vi "JSON to Cluster.vi"(5 "JSON":string, 6 "JSONtext LVClass Serializer in":refnum<class "JSONtext LVClass Serializer.lvclass">, 7 "Item Offset":i32, 8 "error in (no error)":errorcluster, 9 "Element Info":T3(array[cluster]), 10 "Elements":variant[](array[variant]), 11 "ELement Names (as JSON)":string[](array[string])) -> (0 "error out":errorcluster, 3 "Cluster of Variants":variant)   [LabVIEW 2024, in "JSONtext.lvlib"]
uses:
  JSONtext.lvlib
  JSONtext LVClass Serializer.lvclass
  Data Type.ctl
  Tag Type.ctl
  Advance past whitespace.vi
  Commas Needed.vi
  Advance past whitespace and comma.vi
  Advance past next JSON Value (inlined COPY).vi
  Advance past Item Name.vi
  Advance past Line Ending.vi
  Advance past String.vi
  Advance past Number.vi
  Error Cluster From Error Code.vi
  Advance past Array.vi
  Advance past Object.vi
  Parsing Error.vi
  JDP Utility.lvlib
  NI_Data Type.lvlib
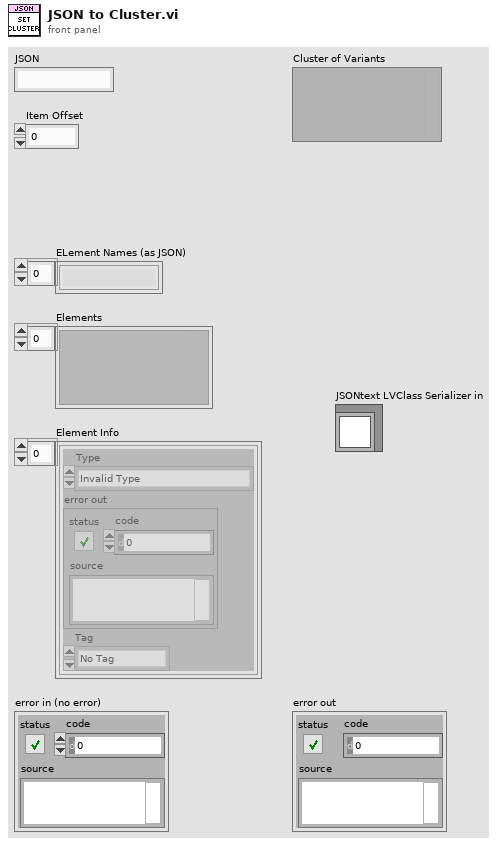
[diagram p1: front panel]
types:
  T1 = typedef "NI_Data Type.lvlib/Data Type.ctl" = enum8{"Invalid Type", "Void", "I8", "I16", "I32", "I64", "U8", "U16", "U32", "U64", "Single Float", "Double Float", "Extended Float", "Single Complex", "Double Complex", "Extended Complex", "Enum U8", "Enum U16", "Enum U32", "Enum U64", "Single Float With Unit", "Double Float With Unit", "Extended Float With Unit", "Single Complex with Unit", "Double Complex with Unit", "Extended Complex with Unit", "Boolean", "String", "Path", "Picture", "Tag", "Array", "Cluster", "Variant", "LV Variant", "Waveform", "Timestamp", "Digital Waveform", "Digital Data", "ExpressData", "Refnum", "External Data", "VI", "Poly VI", "LabVIEW Class Instance", "Fixed Point", "Set Collection", "Map Collection"}
  T2 = typedef "JSONtext.lvlib/Tag Type.ctl" = enum16{"No Tag", "<JSON>", "<JOBJ>", "<UTF8>"}
  T3 = cluster{"Type":T1, "error out":errorcluster, "Tag":T2}[]
  T4 = typedef "JSONtext.lvlib/JSON Value Type.ctl" = enum16{"Not a JSON Value", "JSON Object", "JSON Array", "String", "Number", "true", "false", "null"}
  T5 = typedef "JSONtext.lvlib/Found Items.ctl" = cluster{"Item offset":i32, "Offset past Item":i32, "Name offset":i32, "Offset past Name":i32, "Found":bool, "Item Type":T6, "Item Index":i32, "Start Offset":i32, "Comma Needed For Insert":T7}
  T6 = typedef "JSONtext.lvlib/Parsing State.ctl" = enum16{"Parser Error", "Object", "Array", "String", "Number/Other", "Leading Whitespace", "Object end", "Array end", "Value end"}
  T7 = typedef "JSONtext.lvlib/Comma Needed for Insert.ctl" = enum8{"False", "True", "Following"}
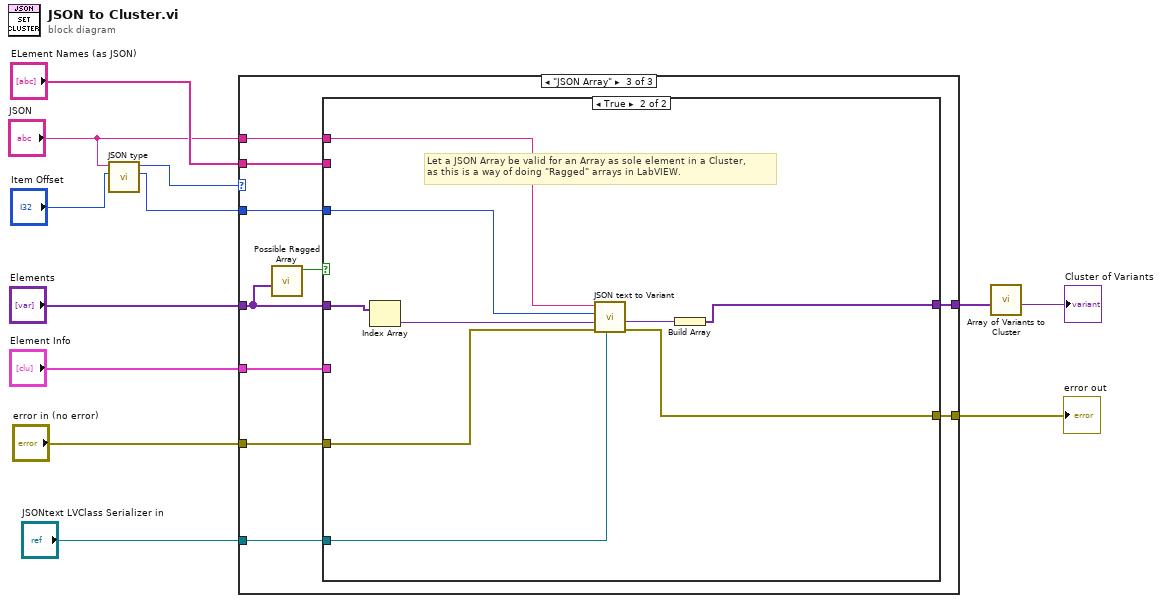
[diagram p0: block diagram]
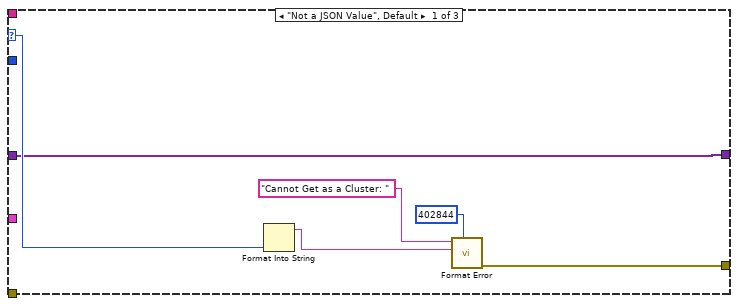
[diagram p2: hidden frame]
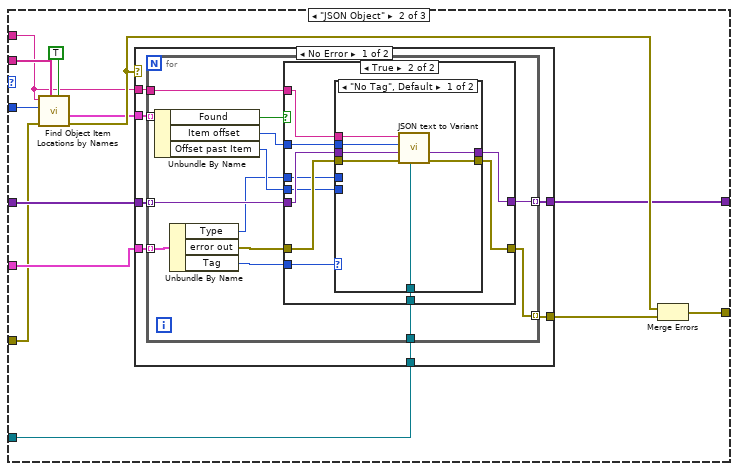
[diagram p3: hidden frame]
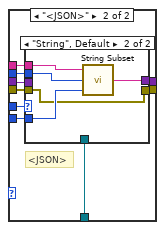
[diagram p5: hidden frame]
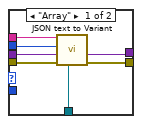
[diagram p6: hidden frame]
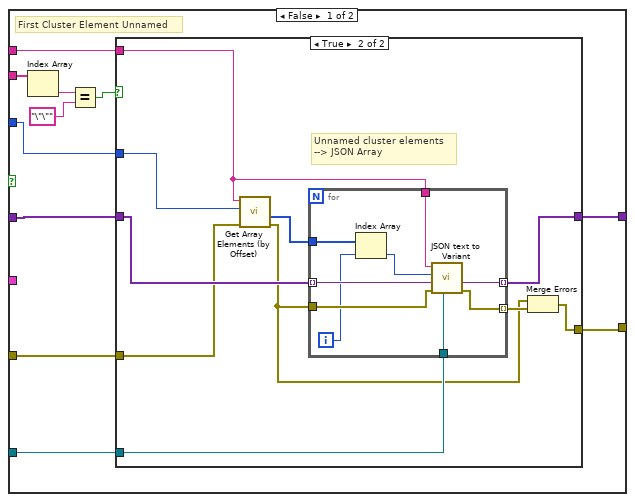
[diagram p8: hidden frame]
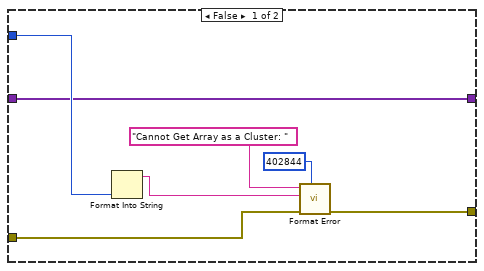
[diagram p9: hidden frame]
diagram:
  n1 = call "JSON type.vi"("Offset"="Item Offset", "JSON"="JSON") -> ("Item Offset"=w4:i32, "JSON Value Type"=w3:T4)  [unwired: 8 in]
  n2 = case shown="\"JSON Array\"" w3 {
    selector: w3 -> [w15 _ _]
    tunnel: "JSONtext LVClass Serializer in" -> [_ w31 w93]
    tunnel: [w13 w21 w100] -> w2
    tunnel: "ELement Names (as JSON)" -> [_ w26 w94]
    tunnel: "Element Info" -> [_ w25 w95]
    tunnel: "Elements" -> [w13 w24 w101]
    tunnel: "error in (no error)" -> [_ w23 w98]
    tunnel: [w14 w22 w99] -> w7
    tunnel: "JSON" -> [_ w20 w97]
    tunnel: w4 -> [_ w19 w96]
    frame "Not a JSON Value", Default {
      n3 = Format Into String(w15) -> (resulting string=w16:string)  [unwired: 3 in, 1 out]
      n4 = call "Format Error.vi"("error code (402842)"=402844, "message part 2"=w16, "error message"="Cannot Get as a Cluster: " ("format string")) -> ("error out"=w14:errorcluster)  [unwired: 8 in]
    }
    frame "JSON Object" {
      n5 = call "Find Object Item Locations by Names.vi"("Insertion point if not found"=TRUE, "Item Names <JSON>"=w26, "error in (no error)"=w23, "Object Offset"=w19, "JSON"=w20) -> ("error out"=w30:errorcluster, "Items"=w28:T5[])  [unwired: 5 in]
      n6 = case shown="No Error" w30 {
        tunnel: [w38 _] -> w27
        tunnel: [w37 w92] -> w21
        tunnel: w25 -> [w36 _]
        tunnel: w28 -> [w35 _]
        tunnel: w24 -> [w34 w92]
        tunnel: w20 -> [w33 _]
        tunnel: w31 -> [w32 _]
        frame No Error {
          n7 = for {
            tunnel: w34 -> [w51] mode=indexing
            tunnel: w33 -> [w50]
            tunnel: [w49] -> w38 mode=indexing
            tunnel: [w48] -> w37 mode=indexing
            tunnel: w36 -> [w47] mode=indexing
            tunnel: w35 -> [w46] mode=indexing
            tunnel: w32 -> [w42]
            n8 = Unbundle By Name(w46) -> ("Found"=w45:bool, "Item offset"=w44:i32, "Offset past Item"=w43:i32)
            n9 = Unbundle By Name(w47) -> ("Type"=w40:T1, "error out"=w41:errorcluster, "Tag"=w39:T2)
            n10 = case shown="True" w45 {
              tunnel: w50 -> [_ w63]
              tunnel: w44 -> [_ w62]
              tunnel: w51 -> [w53 w61]
              tunnel: [w53 w57] -> w48
              tunnel: w41 -> [w52 w60]
              tunnel: [w52 w59] -> w49
              tunnel: w40 -> [_ w58]
              tunnel: w43 -> [_ w55]
              tunnel: w39 -> [_ w56]
              tunnel: w42 -> [_ w54]
              frame False {
              }
              frame True {
                n11 = case shown="\"No Tag\", Default" w56 {
                  tunnel: w63 -> [w70 w79]
                  tunnel: w62 -> [w69 w78]
                  tunnel: w61 -> [w68 w72]
                  tunnel: w60 -> [w67 w74]
                  tunnel: [w66 w73] -> w59
                  tunnel: w58 -> [_ w75]
                  tunnel: [w65 w76] -> w57
                  tunnel: w55 -> [_ w77]
                  tunnel: w54 -> [w64 w71]
                  frame "No Tag", Default {
                    n12 = call "JSON text to Variant.vi"("LVClass Serializer"=w64, "error in (no error)"=w67, "Data Type"=w68, "Offset"=w69, "JSON"=w70) -> ("error out"=w66:errorcluster, "Variant out"=w65:variant)  [unwired: 5 in]
                  }
                  frame "<JSON>" {
                    # "<JSON>"
                    n13 = case shown="\"String\", Default" w75 {
                      tunnel: w79 -> [w86 w91]
                      tunnel: w78 -> [w85 w90]
                      tunnel: w77 -> [_ w89]
                      tunnel: [w82 w88] -> w76
                      tunnel: w74 -> [w83 w87]
                      tunnel: [w81 w87] -> w73
                      tunnel: w72 -> [w84 _]
                      tunnel: w71 -> [w80 _]
                      frame "Array" {
                        n14 = call "JSON text to Variant.vi"("LVClass Serializer"=w80, "error in (no error)"=w83, "Data Type"=w84, "Offset"=w85, "JSON"=w86) -> ("error out"=w81:errorcluster, "Variant out"=w82:variant)  [unwired: 5 in]
                      }
                      frame "String", Default {
                        n15 = call "String Subset.vi"("Offset past End"=w89, "Start offset"=w90, "JSON"=w91) -> ("substring"=w88:string)  [unwired: 2 in]
                      }
                    }
                  }
                }
              }
            }
          }
        }
        frame Error {
          # "Issue 40"
        }
      }
      n16 = Merge Errors(w30, w27) -> (w22:errorcluster)
    }
    frame "JSON Array" {
      n17 = call "Possible Ragged Array.vi"("Array"=w101) -> ("Ragged Array posible"=w102:bool)  [unwired: 10 in]
      n18 = case shown="True" w102 {
        tunnel: w101 -> [w109 w145]
        tunnel: [w107 w146] -> w100
        tunnel: [w112 w144] -> w99
        tunnel: w98 -> [w111 w143]
        tunnel: w97 -> [w110 w142]
        tunnel: w96 -> [w103 w141]
        tunnel: w95 -> [_ _]
        tunnel: w94 -> [w113 _]
        tunnel: w93 -> [w108 w140]
        frame False {
          # "First Cluster Element Unnamed"
          n19 = Index Array(array=w113) -> (element=w105:string)  [unwired: 1 in]
          n20 = Equal?(x=w105, y="\"\"") -> (x = y?=w106:bool)
          n21 = case shown="True" w106 {
            tunnel: [w117 w126] -> w112
            tunnel: w111 -> [w116 w122]
            tunnel: w103 -> [w115 w127]
            tunnel: w110 -> [_ w128]
            tunnel: w109 -> [w114 w123]
            tunnel: [w114 w124] -> w107
            tunnel: w108 -> [_ w125]
            frame False {
              n22 = Format Into String(w115) -> (resulting string=w118:string)  [unwired: 3 in, 1 out]
              n23 = call "Format Error.vi"("error code (402842)"=402844, "error in (no error)"=w116, "message part 2"=w118, "error message"="Cannot Get Array as a Cluster: " ("format string")) -> ("error out"=w117:errorcluster)  [unwired: 7 in]
            }
            frame True {
              # "Unnamed cluster elements\n--> JSON Array"
              n24 = call "Get Array Elements (by Offset).vi"("error in (no error)"=w122, "Offset"=w127, "JSON"=w128) -> ("error out"=w121:errorcluster, "Element Offsets"=w129:i32[])  [unwired: 5 in, 2 out]
              n25 = for {
                tunnel: w123 -> [w139] mode=indexing
                tunnel: w121 -> [w137]
                tunnel: [w136] -> w130 mode=indexing
                tunnel: [w138] -> w124 mode=indexing
                tunnel: w129 -> [w135]
                tunnel: w125 -> [w132]
                tunnel: w128 -> [w131]
                i -> [w133]
                n26 = Index Array(array=w135, index=w133) -> (element=w134:i32)
                n27 = call "JSON text to Variant.vi"("LVClass Serializer"=w132, "error in (no error)"=w137, "Data Type"=w139, "Offset"=w134, "JSON"=w131) -> ("error out"=w136:errorcluster, "Variant out"=w138:variant)  [unwired: 5 in]
              }
              n28 = Merge Errors(w121, w130) -> (w126:errorcluster)
            }
          }
        }
        frame True {
          # "Let a JSON Array be valid for an Array as sole element in a Cluster, \nas this is a way of doing \"Ragged\" arrays in LabVIEW."
          n29 = Index Array(array=w145) -> (element=w148:variant)  [unwired: 1 in]
          n30 = call "JSON text to Variant.vi"("LVClass Serializer"=w140, "error in (no error)"=w143, "Data Type"=w148, "Offset"=w141, "JSON"=w142) -> ("error out"=w144:errorcluster, "Variant out"=w147:variant)  [unwired: 5 in]
          n31 = Build Array(w147) -> (w146:variant[])
        }
      }
    }
  }
  "error out" <- w7
  n32 = call "Array of Variants to Cluster.vi"("Array of Variants"=w2) -> ("Cluster of Variants"=→"Cluster of Variants":variant)  [unwired: 10 in]
